vi "7_Segment_converter.vi"(0 "Time_Format":T2 caption="Time Format") -> (4 "Hours":T1[](array[typedef]), 6 "Min":T1[](array[typedef]), 8 "Sec":T1[](array[typedef]), 10 "ms":T1[](array[typedef]))   [LabVIEW 2023]
uses:
  Controls/7_Segment_Display.ctl
  Controls/Time_Format.ctl
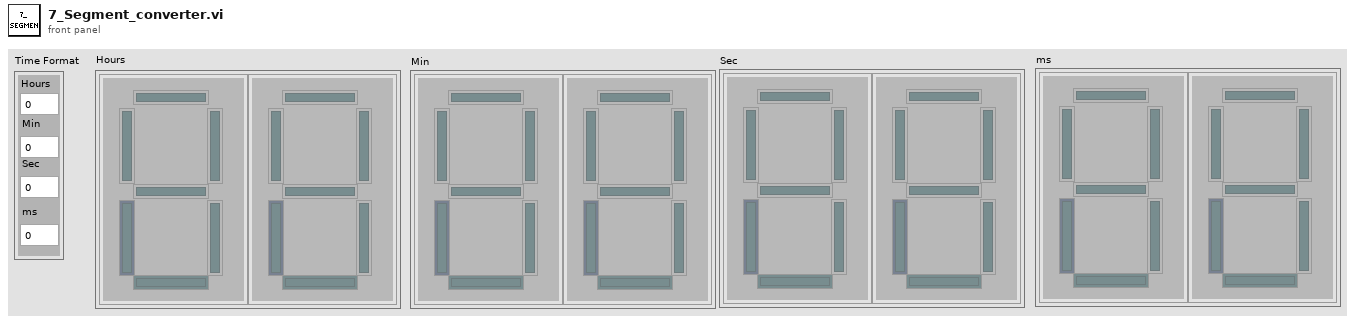
[diagram p1: front panel]
types:
  T1 = typedef "7_Segment_Display.ctl" = cluster{"a":bool, "b":bool, "c":bool, "d":bool, "e":bool, "f":bool, "g":bool}
  T2 = typedef "Time_Format.ctl" = cluster{"Hours":i32, "Min":i32, "Sec":i32, "ms":i32}
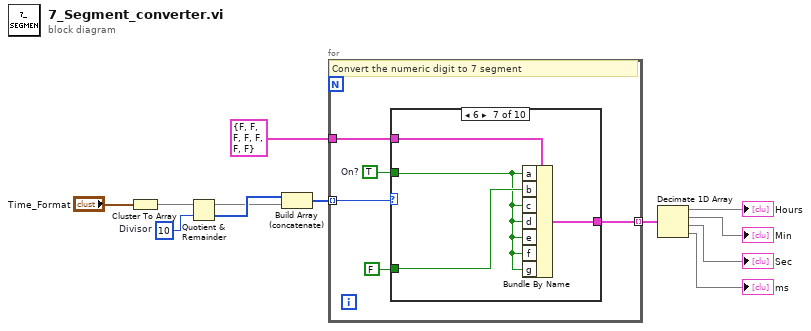
[diagram p0: block diagram]
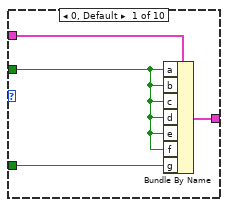
[diagram p2: hidden frame]
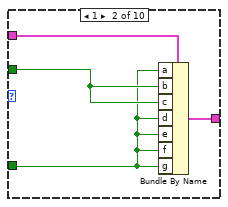
[diagram p3: hidden frame]
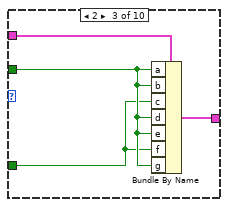
[diagram p4: hidden frame]
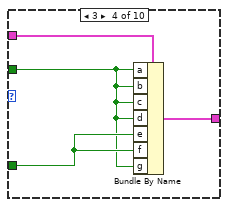
[diagram p5: hidden frame]
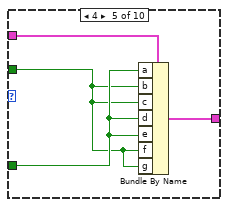
[diagram p6: hidden frame]
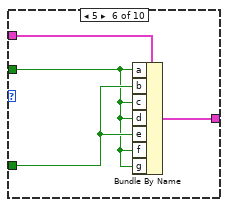
[diagram p7: hidden frame]
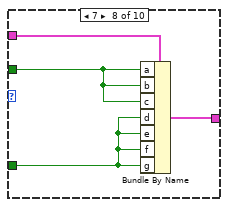
[diagram p8: hidden frame]
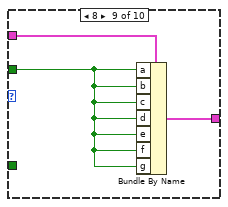
[diagram p9: hidden frame]
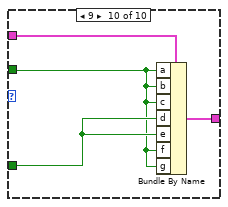
[diagram p10: hidden frame]
diagram:
  w12 = 10  # Divisor
  n1 = Cluster To Array(cluster="Time_Format") -> (array=w10:i32[])
  n2 = Quotient & Remainder(x=w10, y=w12) -> (x-y*floor(x/y)=w5:i32[], floor(x/y)=w6:i32[])
  n3 = Build Array (concatenate)(w6, w5) -> (w7:i32[])
  n4 = for {
    tunnel: w7 -> [w17] mode=indexing
    tunnel: T1 {"a"=FALSE, "b"=FALSE, "c"=FALSE, "d"=FALSE, "e"=FALSE, "f"=FALSE, "g"=FALSE} ("7_Segment") -> [w16]
    tunnel: [w13] -> w8 mode=indexing
    w14 = TRUE  # On?
    # "Convert the numeric digit to 7 segment"
    n5 = case shown="6" w17 {
      tunnel: w16 -> [w21 w25 w29 w33 w37 w41 w45 w49 w52 w56]
      tunnel: FALSE -> [w20 w23 w27 w32 w36 w40 w44 w47 _ w55]
      tunnel: w14 -> [w19 w24 w28 w30 w34 w39 w42 w48 w50 w53]
      tunnel: [w18 w22 w26 w31 w35 w38 w43 w46 w51 w54] -> w13
      frame 0, Default {
        n6 = Bundle By Name(cluster=w21, "a"=w19, "b"=w19, "c"=w19, "d"=w19, "e"=w19, "f"=w19, "g"=w20) -> (w18:T1)
      }
      frame 1 {
        n7 = Bundle By Name(cluster=w25, "a"=w23, "b"=w24, "c"=w24, "d"=w23, "e"=w23, "f"=w23, "g"=w23) -> (w22:T1)
      }
      frame 2 {
        n8 = Bundle By Name(cluster=w29, "a"=w28, "b"=w28, "c"=w27, "d"=w28, "e"=w28, "f"=w27, "g"=w28) -> (w26:T1)
      }
      frame 3 {
        n9 = Bundle By Name(cluster=w33, "a"=w30, "b"=w30, "c"=w30, "d"=w30, "e"=w32, "f"=w32, "g"=w30) -> (w31:T1)
      }
      frame 4 {
        n10 = Bundle By Name(cluster=w37, "a"=w36, "b"=w34, "c"=w34, "d"=w36, "e"=w36, "f"=w34, "g"=w34) -> (w35:T1)
      }
      frame 5 {
        n11 = Bundle By Name(cluster=w41, "a"=w39, "b"=w40, "c"=w39, "d"=w39, "e"=w40, "f"=w39, "g"=w39) -> (w38:T1)
      }
      frame 6 {
        n12 = Bundle By Name(cluster=w45, "a"=w42, "b"=w44, "c"=w42, "d"=w42, "e"=w42, "f"=w42, "g"=w42) -> (w43:T1)
      }
      frame 7 {
        n13 = Bundle By Name(cluster=w49, "a"=w48, "b"=w48, "c"=w48, "d"=w47, "e"=w47, "f"=w47, "g"=w47) -> (w46:T1)
      }
      frame 8 {
        n14 = Bundle By Name(cluster=w52, "a"=w50, "b"=w50, "c"=w50, "d"=w50, "e"=w50, "f"=w50, "g"=w50) -> (w51:T1)
      }
      frame 9 {
        n15 = Bundle By Name(cluster=w56, "a"=w53, "b"=w53, "c"=w53, "d"=w55, "e"=w55, "f"=w53, "g"=w53) -> (w54:T1)
      }
    }
  }
  n16 = Decimate 1D Array(w8) -> (→"Hours":T1[], →"Min":T1[], →"Sec":T1[], →"ms":T1[])
